vi "NumIntegrate_Func_Ch.vi"(11 "Index":i32) -> (3 "Ch":dbl)   [LabVIEW 2019, in "Trajectory_Library.lvlib"]
doc: "Creates a new LINEAR SYSTEM data cluster with the specified values. \n\n\nInputs: \n - XXX -- XXX.\n\nOutputs:\n - XXX -- XXX."
uses:
  Trajectory_Library.lvlib
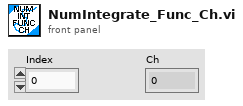
[diagram p1: front panel]
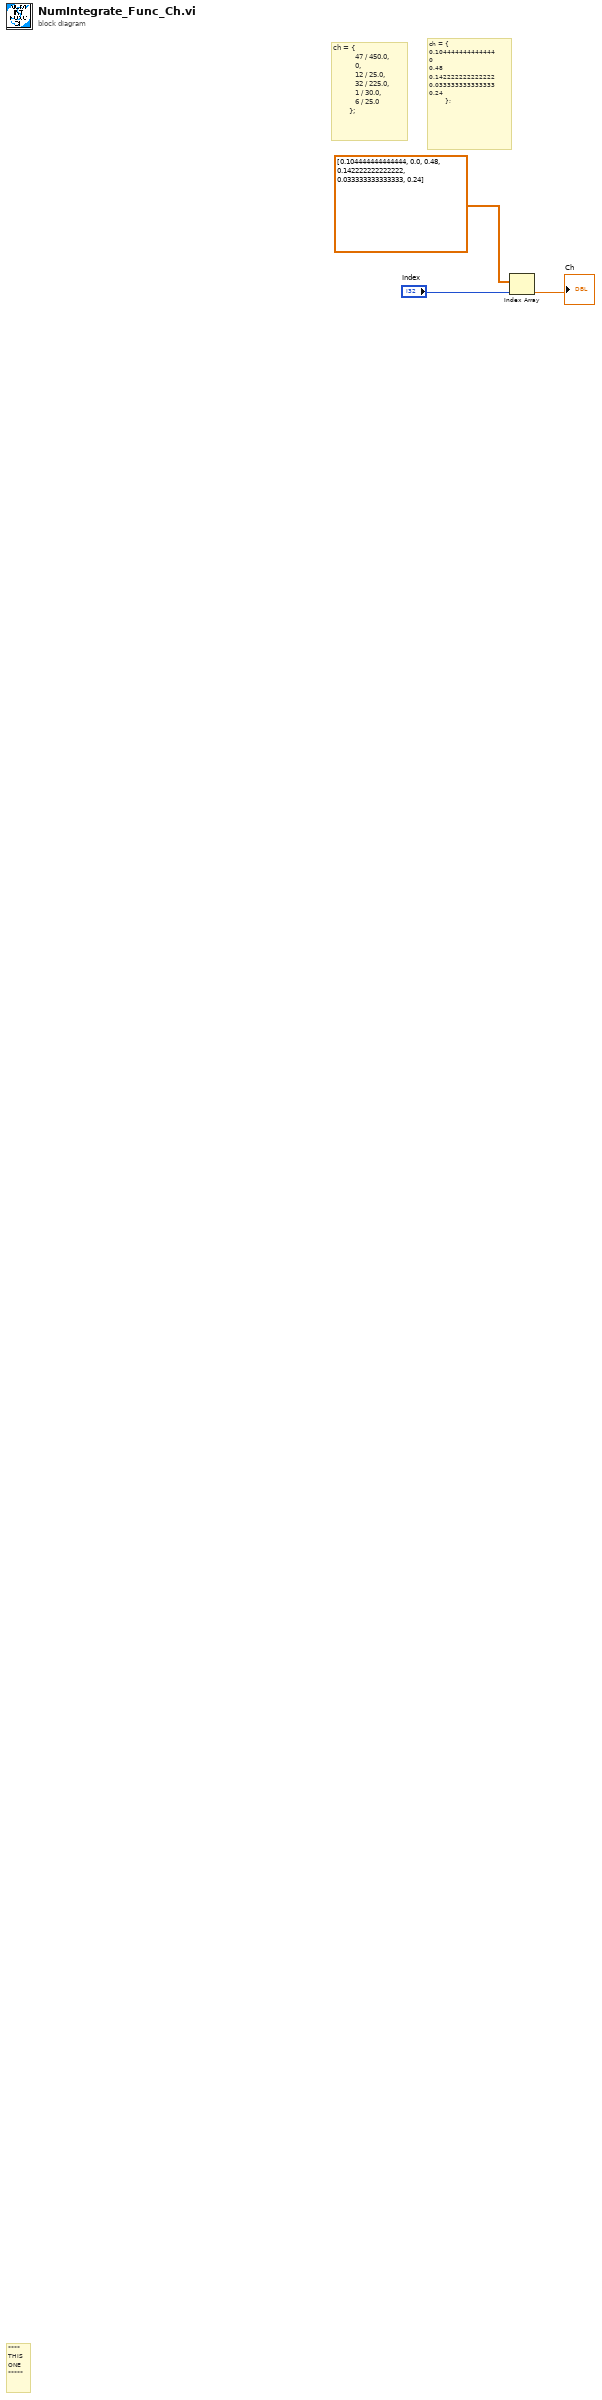
[diagram p0: block diagram]
diagram:
  # "ch = {\n0.104444444444444\n0\n0.48\n0.142222222222222\n0.033333333333333\n0.24\n        };"
  # "ch = {\n           47 / 450.0, \n           0, \n           12 / 25.0, \n           32 / 225.0, \n           1 / 30.0, \n           6 / 25.0\n        };"
  # "****\nTHIS\nONE\n*****"
  n1 = Index Array(array=dbl[] [0.104444444444444, 0.0, 0.48, 0.142222222222222, 0.033333333333333, 0.24], index="Index") -> (element=→"Ch":dbl)
